vi "CRYGet all x_axis.vi"(11 "x_Array in":dbl[](array[numeric])=[1.0, 2.0, 2.0, 3.0, 3.0, 2.0, 2.5, 2.5]) -> (3 "X_axis out":dbl[](array[numeric]))   [LabVIEW 2013]
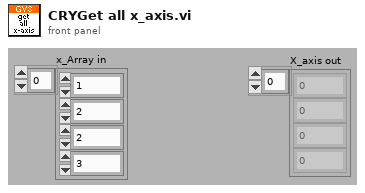
[diagram p1: front panel]
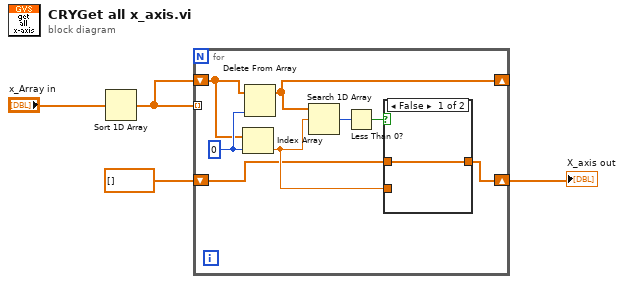
[diagram p0: block diagram]
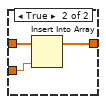
[diagram p2: hidden frame]
diagram:
  n1 = Sort 1D Array(array="x_Array in") -> (sorted array=w2:dbl[])
  n2 = for {
    tunnel: w2 -> [_] mode=indexing
    shift-right: [w5] -> _
    shift-left: w2 -> [w11]
    shift-right: [w6] -> w1
    shift-left: dbl[] [] ("sorted array") -> [w7]
    w12 = 0 ("index")
    n3 = Index Array(array=w11, index=w12) -> (element=w8:dbl)
    n4 = Delete From Array(array=w11, index=w12) -> (array with subset deleted=w5:dbl[])  [unwired: 1 in, 1 out]
    n5 = Search 1D Array(1D array=w5, element=w8) -> (index of element=w9:i32)  [unwired: 1 in]
    n6 = Less Than 0?(x=w9) -> (x < 0?=w10:bool)
    n7 = case shown="False" w10 {
      tunnel: w8 -> [_ w16]
      tunnel: w7 -> [w13 w15]
      tunnel: [w13 w14] -> w6
      frame False {
      }
      frame True {
        n8 = Insert Into Array(array=w15, new element=w16) -> (w14:dbl[])  [unwired: 1 in]
      }
    }
  }
  "X_axis out" <- w1
